vi "NumOfUsed.vi"(8 "error in (no error)":errorcluster, 11 "worksheet_Refnum":refnum<k7>) -> (0 "error out":errorcluster, 1 "Rows(0)":i32, 2 "Columns(0)":i32, 3 "worksheet_Refnum":refnum<k7>)   [LabVIEW 2015]
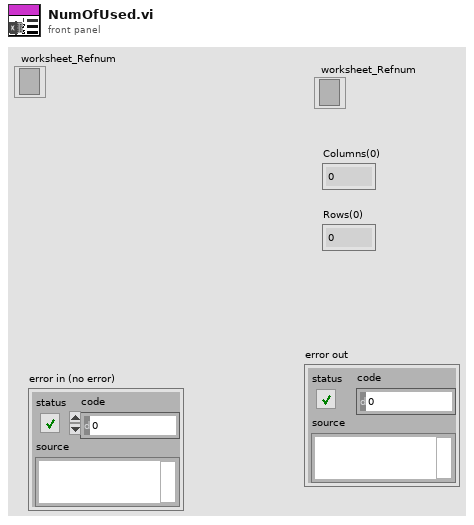
[diagram p1: front panel]
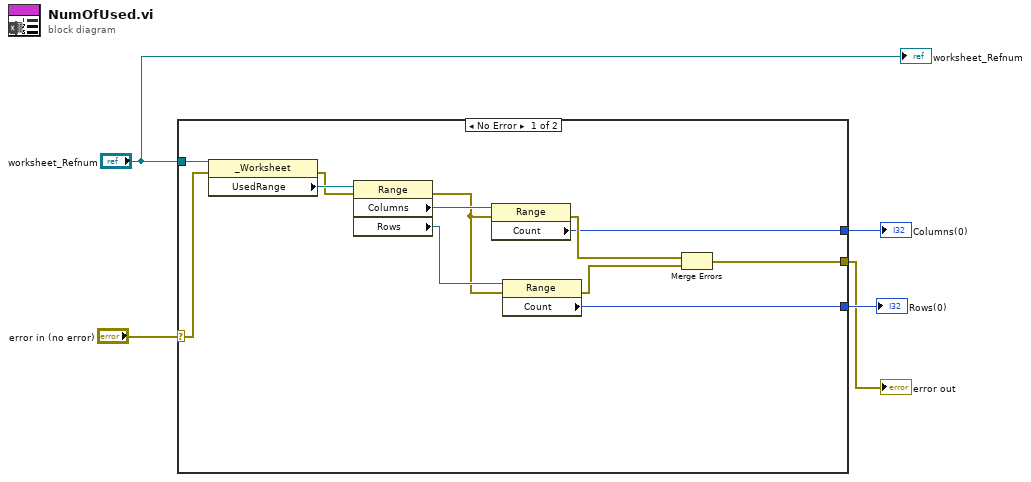
[diagram p0: block diagram]
diagram:
  n1 = case shown="No Error" "error in (no error)" {
    selector: "error in (no error)" -> [w13 w18]
    tunnel: [w16 _] -> w5
    tunnel: [w6 _] -> w1
    tunnel: [w8 w18] -> w3
    tunnel: "worksheet_Refnum" -> [w7 _]
    frame No Error {
      n2 = property class="_Worksheet"(reference=w7, error in=w13) -> (error out=w12:errorcluster, "UsedRange"=w14:refnum<k7>)  [unwired: 1 out]
      n3 = property class="Range"(reference=w14, error in=w12) -> (error out=w11:errorcluster, "Columns"=w15:refnum<k7>, "Rows"=w17:refnum<k7>)  [unwired: 1 out]
      n4 = property class="Range"(reference=w15, error in=w11) -> (error out=w10:errorcluster, "Count"=w6:i32)  [unwired: 1 out]
      n5 = property class="Range"(reference=w17, error in=w11) -> (error out=w9:errorcluster, "Count"=w16:i32)  [unwired: 1 out]
      n6 = Merge Errors(w10, w9) -> (w8:errorcluster)
    }
    frame Error {
    }
  }
  "Columns(0)" <- w1
  "Rows(0)" <- w5
  "error out" <- w3
  "worksheet_Refnum" <- "worksheet_Refnum"
